vi "ABPW Enthalpy BackWardof f Pure Water (K).vi"(1 "Presssure (Pa)":dbl[unit], 2 "SEPW (J/kg)":dbl[unit]) -> (0 "Tc":dbl[unit])   [LabVIEW 2018]
panel:
  out "Temprature of Pure Water \nKelvin Degree":dbl[unit](slide) scale=273.0..373.0
  out "Tk":dbl[unit]
  out "Temprature of Pure Water\nCentigrade Degree":dbl[unit](slide) scale=0.0..100.0
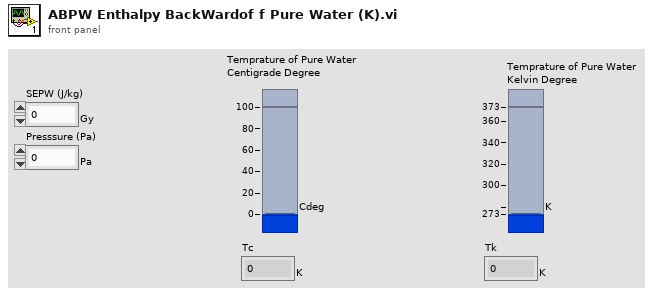
[diagram p1: front panel]
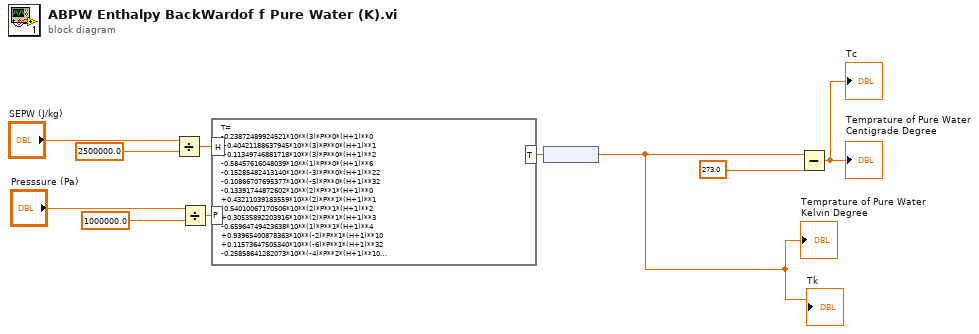
[diagram p0: block diagram]
diagram:
  n1 = Divide(x="SEPW (J/kg)", y=dbl[unit] 2500000.0) -> (x/y=w10:dbl)
  n2 = Divide(x="Presssure (Pa)", y=dbl[unit] 1000000.0) -> (x/y=w7:dbl)
  n3 = formula code="T=\n-0.23872489924521*10**(3)*P**0*(H+1)**0\n+0.40421188637945*10**(3)*P**0*(H+1)**1\n+0.11349746881718*10**(3)*P**0*(H+1)**2\n-0.58457616048039*10**(1)*P**0*(H+1)**6\n-0.15285482413140*10**(-3)*P**0*(H+1)**22\n-0.10866707695377*10**(-5)*P**0*(H+1)**32\n-0.13391744872602*10**(2)*P**1*(H+1)**0\n+0.43211039183559*10**(2)*P**1*(H+1)**1\n-0.54010067170506*10**(2)*P**1*(H+1)**2\n+0.30535892203916*10**(2)*P**1*(H+1)**3\n-0.65964749423638*10**(1)*P**1*(H+1)**4\n+0.93965400878363*10**(-2)*P**1*(H+1)**10\n+0.11573647505340*10**(-6)*P**1*(H+1)**32\n-0.25858641282073*10**(-4)*P**2*(H+1)**10\n-0.40644363084799*10**(-8)*P**2*(H+1)**32\n+0.66456186191635*10**(-7)*P**3*(H+1)**10\n+0.80670734103027*10**(-10)*P**3*(H+1)**32\n-0.93477771213947*10**(-12)*P**4*(H+1)**32\n+0.58265442020601*10**(-14)*P**5*(H+1)**32\n-0.15020185953503*10**(-16)*P**6*(H+1)**32;"("H"=w10, "P"=w7) -> ("T"=w6:dbl)
  n4 = node(w6) -> (w2:dbl[unit])
  "Tk" <- w2
  "Temprature of Pure Water \nKelvin Degree" <- w2
  n5 = Subtract(x=w2, y=dbl[unit] 273.0) -> (x-y=→"Temprature of Pure Water\nCentigrade Degree" →"Tc":dbl[unit])
